vi "Untitled 8.vi"() -> ()   [LabVIEW 2019]
panel:
  out "XY Graph":cluster{i32[], dbl[]}(graph)
  in  "theta_min":dbl
  in  "C":dbl
  in  "B":dbl
  in  "A":dbl
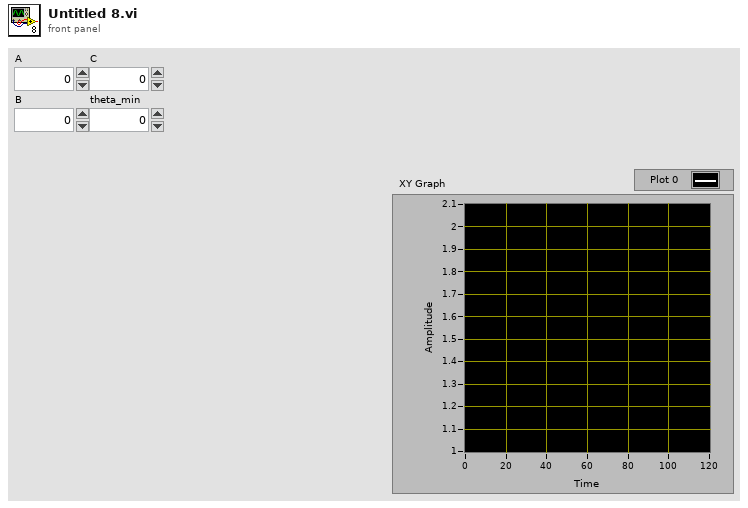
[diagram p1: front panel]
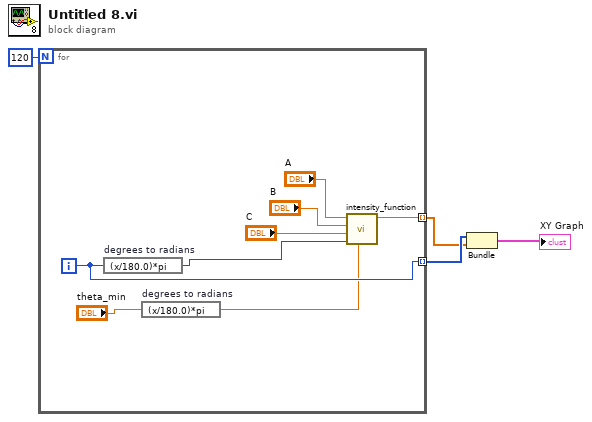
[diagram p0: block diagram]
diagram:
  n1 = for {
    N: 120 -> [_]
    tunnel: [w9] -> w2 mode=indexing
    tunnel: [w7] -> w3 mode=indexing
    i -> [w7]
    n2 = expression code="(x/180.0)*pi" "degrees to radians"(w7) -> (w8:i32)
    n3 = expression code="(x/180.0)*pi" "degrees to radians"("theta_min") -> (w5:dbl)
    n4 = call "intensity_function.vi"("theta_min"=w5, "theta"=w8, "C"="C", "B"="B", "A"="A") -> ("output variable"=w9:dbl)  [unwired: 6 in]
  }
  n5 = Bundle(w3, w2) -> (→"XY Graph":cluster{i32[], dbl[]})  [unwired: 1 in]
